vi "Test - Draw Line 1.vi"() -> ()   [LabVIEW 2020, in "Raster (FPGA).lvlib"]
uses:
  Raster (FPGA).lvlib
  Point 2D (I32).ctl
  Libraries/Utility/Utility.lvlib
  Rectangle Dimensions.ctl
panel:
  out "new picture":picture
  out "Pixel Data out":u32[][](array[colorbox])
  # "(0,0)"
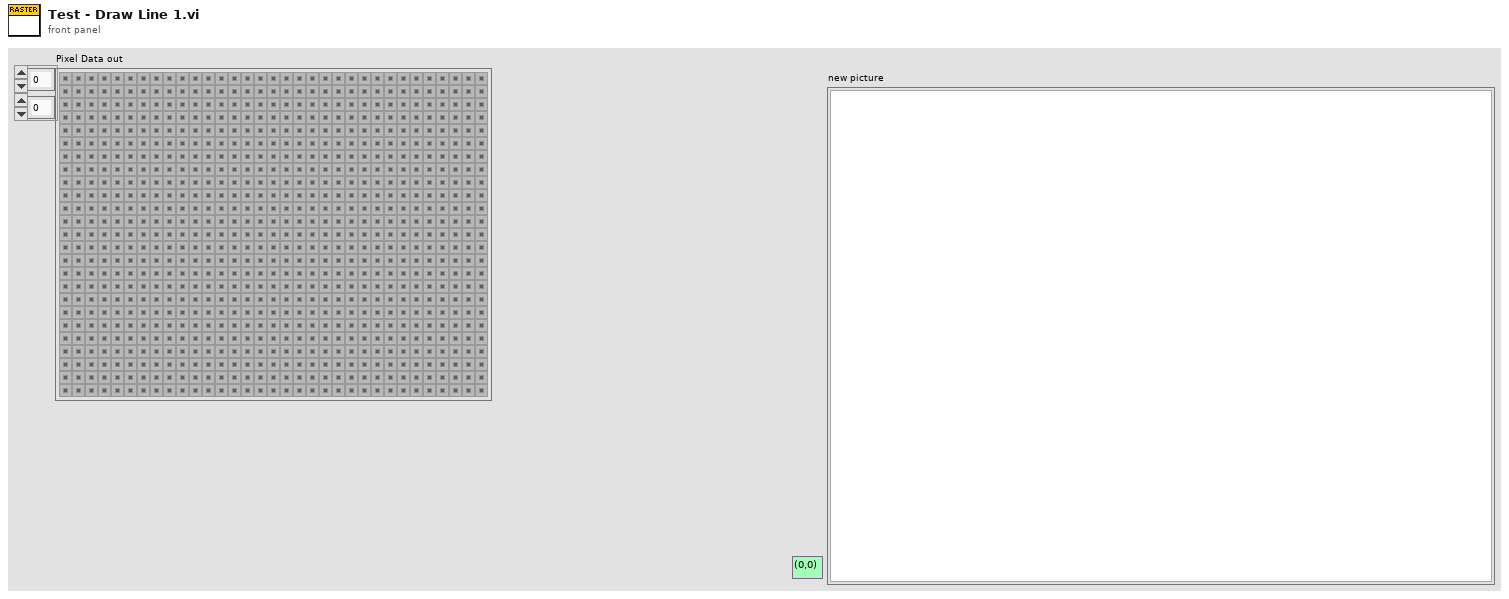
[diagram p1: front panel]
types:
  T1 = typedef "Raster (FPGA).lvlib/Rectangle Dimensions.ctl" = cluster{"Width":u32, "Height":u32}
  T2 = typedef "Raster (FPGA).lvlib/Point 2D (I32).ctl" = cluster{"x":i32, "y":i32}
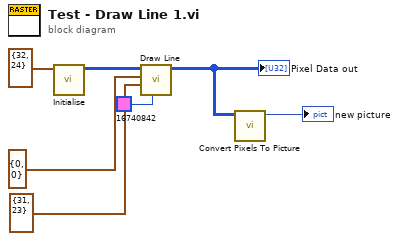
[diagram p0: block diagram]
diagram:
  n1 = call "Initialise.vi"("Screen Dimensions"=T1 {"Width"=32, "Height"=24}) -> ("Pixel Data out"=w7:u32[][])  [unwired: 10 in]
  n2 = call "Draw Line.vi"("Colour"=u32 16740842, "Point 2"=T2 {"x"=31, "y"=23} ("Point 1"), "Point 1"=T2 {"x"=0, "y"=0}, "Pixel Data in"=w7) -> ("Pixel Data out"=w3:u32[][])  [unwired: 7 in]
  "Pixel Data out" <- w3
  n3 = call "Convert Pixels To Picture.vi"("Pixel Data in"=w3) -> ("2D Picture"=→"new picture":picture)  [unwired: 9 in, 1 out]
